vi "RVC 3D Transformation.vi"() -> ()   [LabVIEW 2013]
uses:
  <vilib>/robotics/Kinematics/RotateX.vi
  <vilib>/robotics/Kinematics/RotateY.vi
  <vilib>/robotics/Kinematics/RotateZ.vi
  <vilib>/Analysis/baseanly.llb/A x B.vi
  <vilib>/Analysis/baseanly.llb/Real A x B.vi
  <vilib>/robotics/Kinematics/NI_Kinematics.lvlib
panel:
  out "transformation matrix":picture
  in  "Position":dbl[](array[numeric])=[1.0, 1.0, 1.0]
  in  "angles":cluster{"roll":dbl, "pitch":dbl, "yaw":dbl}={"roll"=1.0, "pitch"=1.0, "yaw"=1.0} {"roll" scale=-3.14..3.14; "pitch" scale=-3.14..3.14; "yaw" scale=-1.54..1.54}
  out "3D Picture":refnum<vi>(3d-picture)
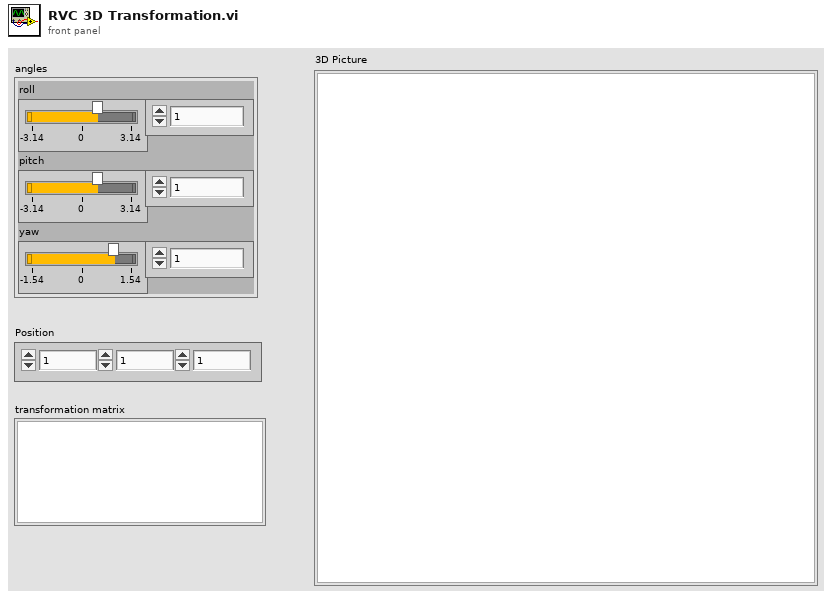
[diagram p1: front panel]
types:
  T1 = typedef "NI_Matrix.lvlib/RealMatrix.ctl" = dbl[][]
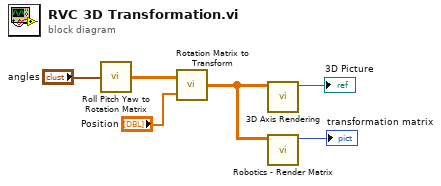
[diagram p0: block diagram]
diagram:
  n1 = call <vilib>:"Roll Pitch Yaw to Rotation Matrix.vi"("angles"="angles") -> ("rotation matrix"=w2:T1)
  n2 = call <vilib>:"Rotation Matrix to Transform.vi"("translation vector"="Position", "rotation matrix"=w2) -> ("transform"=w1:T1)
  n3 = call "3D Axis Rendering.vi"("rotation matrix"=w1) -> ("SceneNode out"=→"3D Picture":refnum<vi>)  [unwired: 9 in, 1 out]
  n4 = call "Robotics - Render Matrix.vi"("A"=w1) -> ("picture out"=→"transformation matrix":picture)  [unwired: 10 in]
